vi "PointInOval.vi"(1 "rect":T1 caption="矩形", 2 "point":cluster{"x":i16, "y":i16} caption="点") -> (0 "pt in oval":bool caption="椭圆中的点")   [LabVIEW 2012, in "Picture Box Tools.lvlib" / "Rect Tools.lvlib"]
uses:
  Rect Tools.lvlib
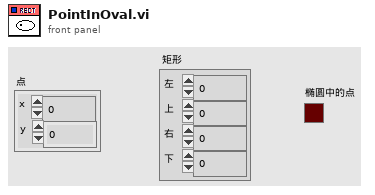
[diagram p1: front panel]
types:
  T1 = cluster{"left":i16, "top":i16, "right":i16, "bottom":i16}
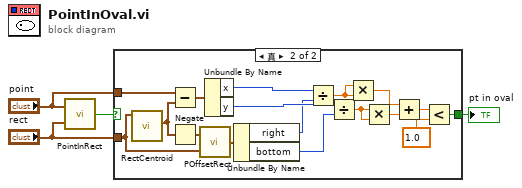
[diagram p0: block diagram]
diagram:
  n1 = call <vilib>:"PointInRect.vi"("rect"="rect", "point"="point") -> ("pt in rect"=w3:bool)
  n2 = case shown="真" w3 {
    selector: w3 -> [w5 _]
    tunnel: [w5 w7] -> w4
    tunnel: "rect" -> [_ w20]
    tunnel: "point" -> [_ w22]
    frame False {
    }
    frame True {
      n3 = call "RectCentroid.vi"("Rect In"=w20) -> ("point"=w21:cluster{"x":i16, "y":i16})  [unwired: 8 in, 2 out]
      n4 = Subtract(x=w22, y=w21) -> (x-y=w18:cluster{"x":i16, "y":i16})
      n5 = Negate(x=w21) -> (-x=w6:cluster{"x":i16, "y":i16})
      n6 = call <vilib>:"POffsetRect.vi"("rect"=w20, "point"=w6) -> ("offset rect"=w19:T1)
      n7 = Unbundle By Name(w18) -> ("x"=w17:i16, "y"=w16:i16)
      n8 = Unbundle By Name(w19) -> ("right"=w15:i16, "bottom"=w14:i16)
      n9 = Divide(x=w17, y=w15) -> (x/y=w13:dbl)
      n10 = Divide(x=w16, y=w14) -> (x/y=w12:dbl)
      n11 = Multiply(x=w13, y=w13) -> (x*y=w11:dbl)
      n12 = Multiply(x=w12, y=w12) -> (x*y=w10:dbl)
      n13 = Add(x=w11, y=w10) -> (x+y=w9:dbl)
      n14 = Less?(x=w9, y=1.0) -> (x < y?=w7:bool)
    }
  }
  "pt in oval" <- w4
